vi "TransmitString.vi"(8 "error in (no error)":errorcluster, 9 "lock semaphore":bool, 10 "string to transmit":string, 11 "queue cluster":T1) -> (0 "error out":errorcluster, 3 "queue cluster out":T1)   [LabVIEW 2014]
uses:
  typedefs/QueueCluster.ctl
  typedefs/clientStatus.ctl
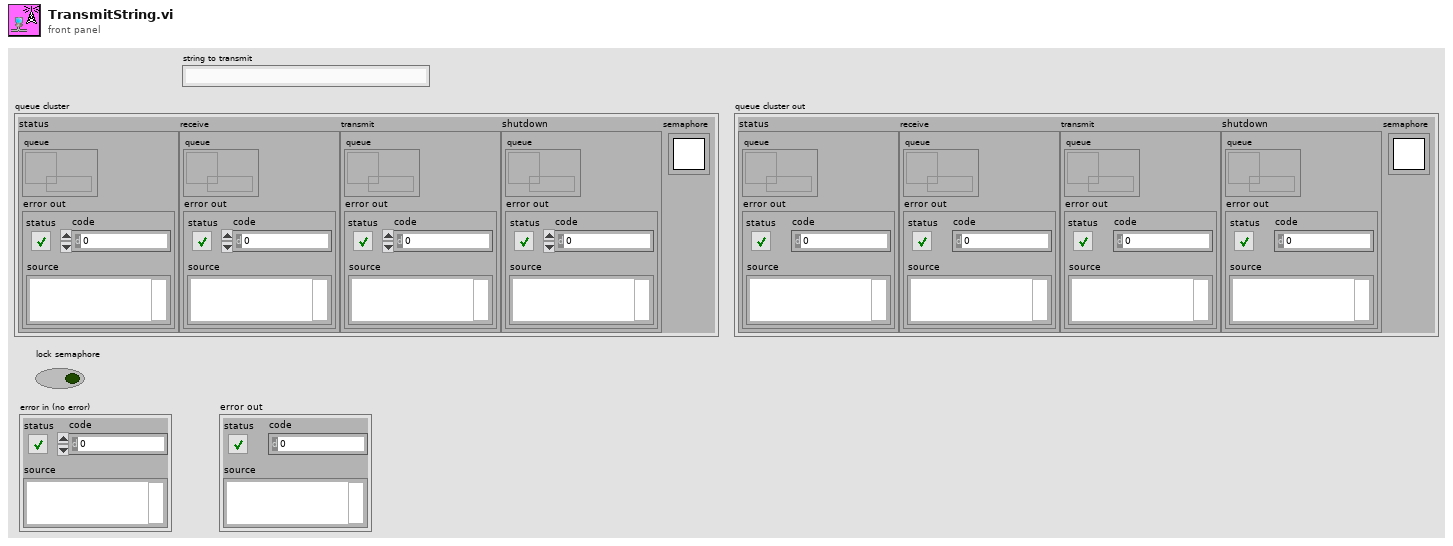
[diagram p1: front panel]
types:
  T1 = typedef "QueueCluster.ctl" = cluster{"status":cluster{"queue":refnum<queue>, "error out":errorcluster}, "receive":cluster{"queue":refnum<queue>, "error out":errorcluster}, "transmit":cluster{"queue":refnum<queue>, "error out":errorcluster}, "shutdown":cluster{"queue":refnum<queue>, "error out":errorcluster}, "semaphore":T2}
  T2 = typedef "Semaphore RefNum" = refnum<k1>
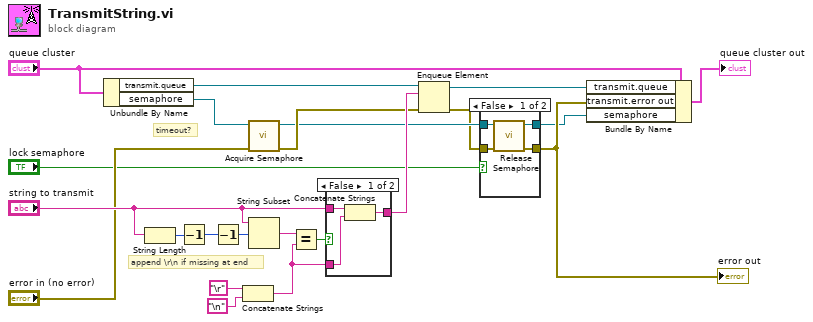
[diagram p0: block diagram]
diagram:
  # "timeout?"
  # "append \\r\\n if missing at end"
  n1 = Unbundle By Name("queue cluster") -> ("transmit.queue"=w22:refnum<queue>, "semaphore"=w8:T2)
  n2 = String Length(string="string to transmit") -> (length=w18:i32)
  n3 = Decrement(x=w18) -> (x-1=w17:i32)
  n4 = Decrement(x=w17) -> (x-1=w11:i32)
  n5 = Concatenate Strings("\r", "\n") -> (w10:string)
  n6 = call <vilib>:"Acquire Semaphore.vi"("error in (no error)"="error in (no error)", "semaphore"=w8) -> ("error out"=w6:errorcluster, "semaphore out"=w5:T2)  [unwired: 3 in, 1 out]
  n7 = String Subset(string="string to transmit", offset (0)=w11) -> (substring=w16:string)  [unwired: 1 in]
  n8 = Equal?(x=w16, y=w10) -> (x = y?=w15:bool)
  n9 = case shown="False" w15 {
    tunnel: "string to transmit" -> [w24 w26]
    tunnel: [w25 w26] -> w13
    tunnel: w10 -> [w23 _]
    frame False {
      n10 = Concatenate Strings(w24, w23) -> (w25:string)
    }
    frame True {
    }
  }
  n11 = Enqueue Element(queue=w22, element=w13, error in (no error)=w6) -> (queue out=w19:refnum<queue>, error out=w4:errorcluster)  [unwired: 1 in, 1 out]
  n12 = case shown="False" "lock semaphore" {
    tunnel: w5 -> [w30 w32]
    tunnel: w4 -> [w29 w31]
    tunnel: [w28 w31] -> w3
    tunnel: [w27 w32] -> w2
    frame False {
      n13 = call <vilib>:"Release Semaphore.vi"("error in (no error)"=w29, "semaphore"=w30) -> ("error out"=w28:errorcluster, "semaphore out"=w27:T2)  [unwired: 4 in]
    }
    frame True {
    }
  }
  "error out" <- w3
  n14 = Bundle By Name(cluster="queue cluster", "transmit.queue"=w19, "transmit.error out"=w3, "semaphore"=w2) -> (→"queue cluster out":T1)
